vi "Measurement Parser.vi"(8 "error in (no error)":errorcluster, 9 "Generic Card in":refnum<class "Generic Card.lvclass">, 10 "Data Array":dbl[](array[numeric]), 11 "Tektronix DMM4020 in":refnum<class "Tektronix DMM4020.lvclass">) -> (0 "error out":errorcluster, 2 "Waveform Graph":dynamicdata(graph), 3 "Tektronix DMM4020 out":refnum<class "Tektronix DMM4020.lvclass">)   [LabVIEW 2014, in "Generic Power Analyzer.lvlib" / "Tektronix DMM4020.lvlib" / "Tektronix DMM4020.lvclass"]
uses:
  Tektronix DMM4020.lvclass
  Generic Instrument/Generic Card/Generic Card.lvclass
  Generic Power Analyzer/Generic Power Analyzer.lvclass
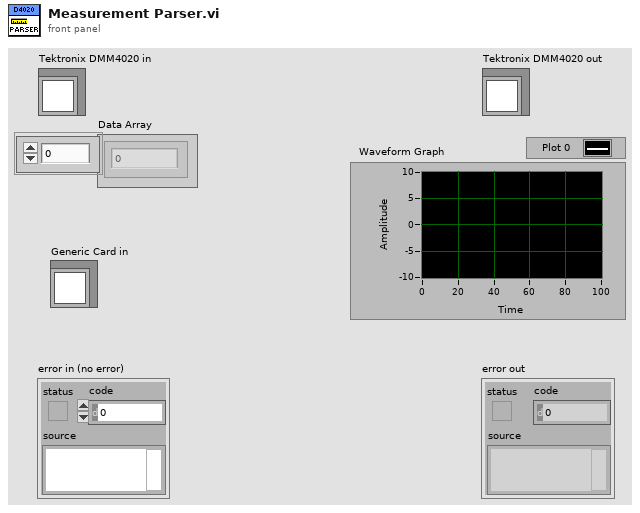
[diagram p1: front panel]
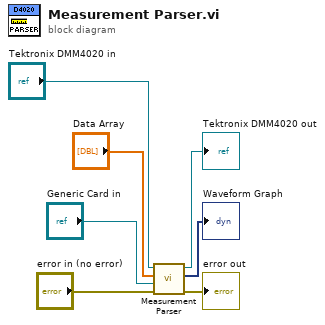
[diagram p0: block diagram]
diagram:
  n1 = call-parent "Measurement Parser.vi"("error in (no error)"="error in (no error)", "Generic Card in"="Generic Card in", "Data Array"="Data Array", "Generic Power Analyzer in"="Tektronix DMM4020 in") -> ("error out"=→"error out":errorcluster, "Waveform Graph"=→"Waveform Graph":dynamicdata, "Generic Power Analyzer out"=→"Tektronix DMM4020 out":refnum<class "Tektronix DMM4020.lvclass">)  [unwired: 5 in]
